vi "AlarmCreateOrUpdateTrendRulesRoutedMessage_Parse.vi"(8 "error in (no error)":errorcluster, 11 "Message":T8) -> (0 "error out":errorcluster, 1 "Body":T1, 2 "Header":T7, 3 "AlarmCreateOrUpdateTrendRulesRoutedMessage":T6)   [LabVIEW 2017]
uses:
  <vilib>/addons/InsightCM/MessageBus/Base/controls/Message.ctl
  <vilib>/addons/InsightCM/MessageBus/Base/controls/MessageHeader.ctl
  <vilib>/addons/InsightCM/MessageBus/Base/controls/KeyValuePair.ctl
  <vilib>/addons/InsightCM/MessageBus/MessageLibrary/TrendAlarm/controls/AlarmCreateOrUpdateTrendRulesRoutedMessage.ctl
  <vilib>/addons/InsightCM/MessageBus/MessageLibrary/TrendAlarm/controls/AlarmCreateOrUpdateTrendRulesRoutedMessageBody.ctl
  <vilib>/addons/InsightCM/MessageBus/Base/controls/TrendAlarmRule.ctl
  <vilib>/addons/InsightCM/MessageBus/Base/controls/TrendAlarmLevel.ctl
  <vilib>/addons/InsightCM/MessageBus/Base/controls/AlarmAction.ctl
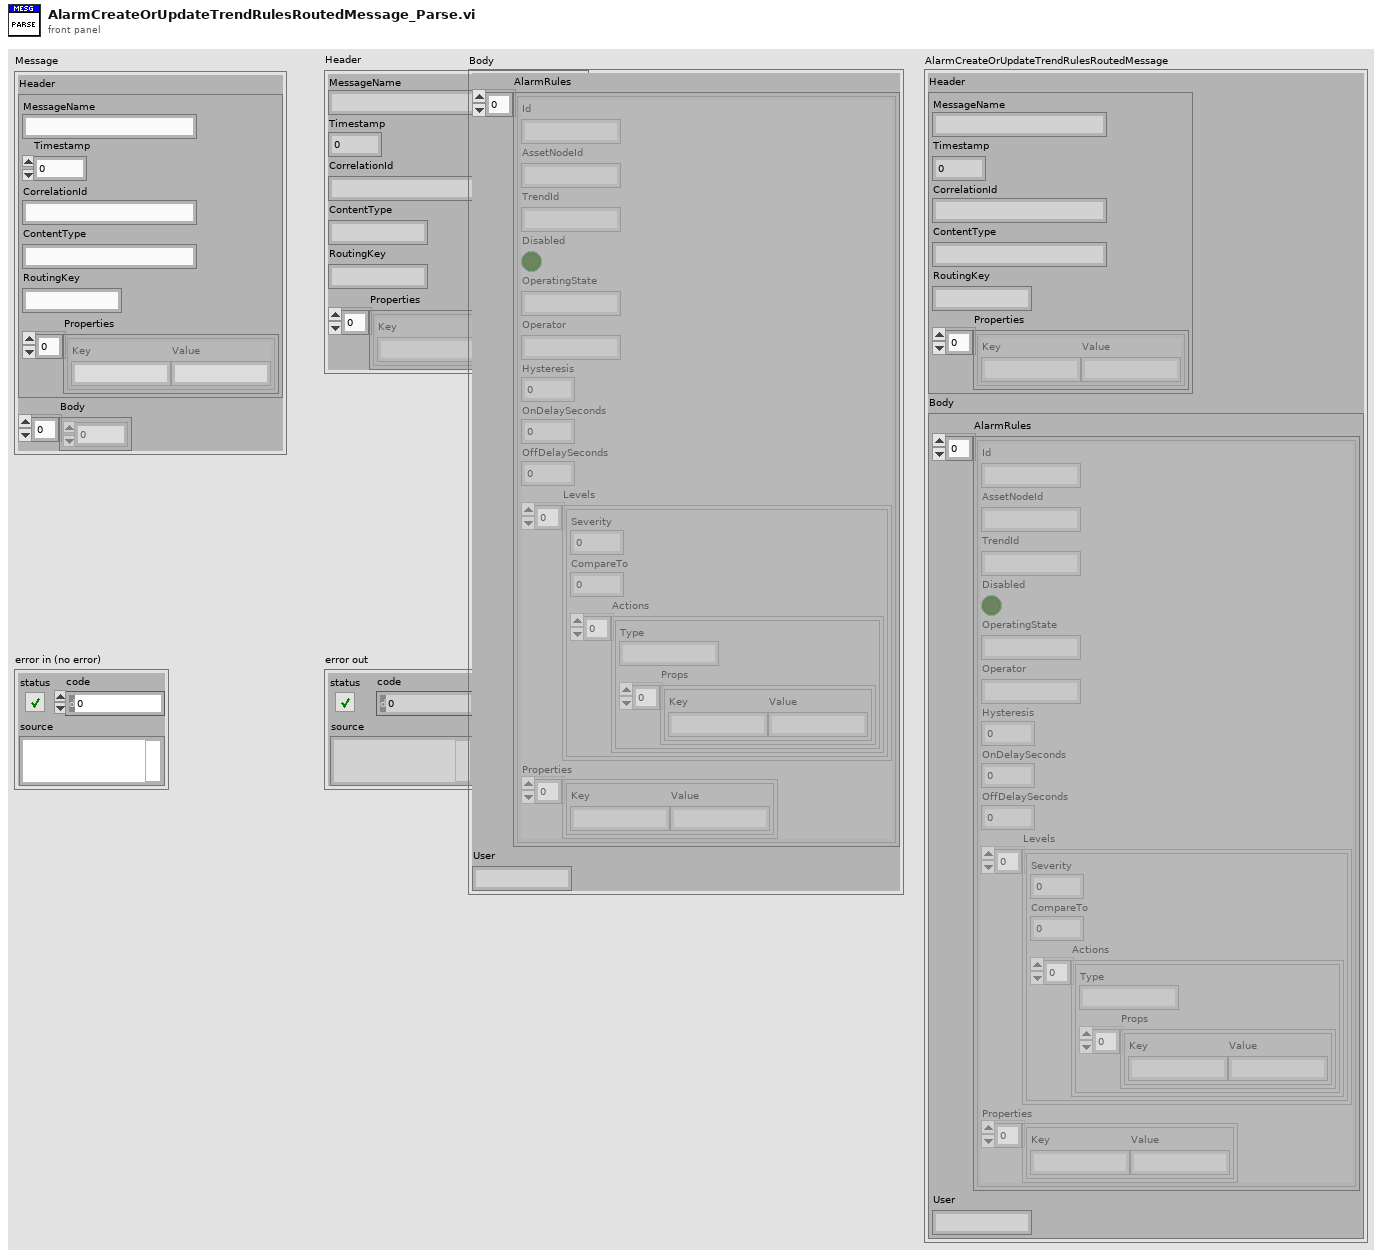
[diagram p1: front panel]
types:
  T1 = typedef "AlarmCreateOrUpdateTrendRulesRoutedMessageBody.ctl" = cluster{"AlarmRules":T2[], "User":string}
  T2 = typedef "TrendAlarmRule.ctl" = cluster{"Id":string, "AssetNodeId":string, "TrendId":string, "Disabled":bool, "OperatingState":string, "Operator":string, "Hysteresis":dbl, "OnDelaySeconds":dbl, "OffDelaySeconds":dbl, "Levels":T3[], "Properties":T5[]}
  T3 = typedef "TrendAlarmLevel.ctl" = cluster{"Severity":i32, "CompareTo":dbl, "Actions":T4[]}
  T4 = typedef "AlarmAction.ctl" = cluster{"Type":string, "Props":T5[]}
  T5 = typedef "KeyValuePair.ctl" = cluster{"Key":string, "Value":string}
  T6 = typedef "AlarmCreateOrUpdateTrendRulesRoutedMessage.ctl" = cluster{"Header":T7, "Body":T1}
  T7 = typedef "MessageHeader.ctl" = cluster{"MessageName":string, "Timestamp":i64, "CorrelationId":string, "ContentType":string, "RoutingKey":string, "Properties":T5[]}
  T8 = typedef "Message.ctl" = cluster{"Header":T7, "Body":u8[]}
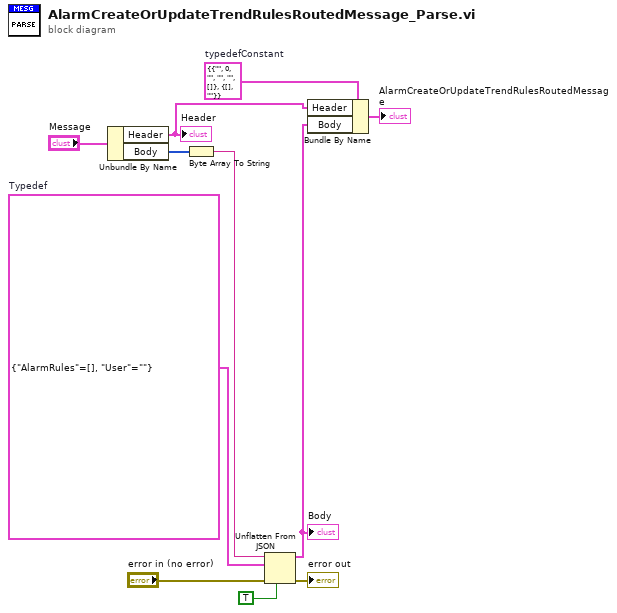
[diagram p0: block diagram]
diagram:
  w3 = T6 {"Header"={"MessageName"="", "Timestamp"=0, "CorrelationId"="", "ContentType"="", "RoutingKey"="", "Properties"=[]}, "Body"={"AlarmRules"=[], "User"=""}}  # typedefConstant
  w7 = T1 {"AlarmRules"=[], "User"=""}  # Typedef
  n1 = Unbundle By Name("Message") -> ("Header"=w9:T7, "Body"=w1:u8[])
  "Header" <- w9
  n2 = Byte Array To String(unsigned byte array=w1) -> (string=w6:string)
  n3 = Unflatten From JSON(JSON string=w6, type and defaults=w7, default null elements? (F)=TRUE, error in (no error)="error in (no error)") -> (value=w5:T1, error out=→"error out":errorcluster)  [unwired: 3 in]
  "Body" <- w5
  n4 = Bundle By Name(cluster=w3, "Header"=w9, "Body"=w5) -> (→"AlarmCreateOrUpdateTrendRulesRoutedMessage":T6)
